vi "Configure System (Beeper).vi"(8 "error in (no error)":errorcluster, 9 "Beeper Tone (3: Tone 3)":u16(ring)=3 items=["Tone 1"=1, "Tone 2"=2, "Tone 3"=3, "Tone 4"=4, "Tone 5"=5], 10 "Beeper State (F:Disable)":bool, 11 "VISA resource name":refnum<visa-resource-name>) -> (0 "error out":errorcluster, 3 "VISA resource name out":refnum<visa-resource-name>)   [LabVIEW 2017, in "Agilent E4980.lvlib"]
doc: "Enables or disables a beeper sound, and selects a beeper sound tone."
uses:
  Agilent E4980.lvlib
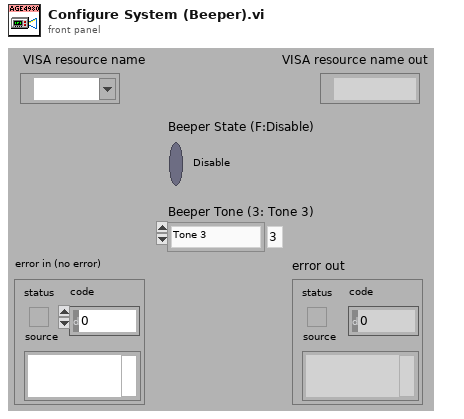
[diagram p1: front panel]
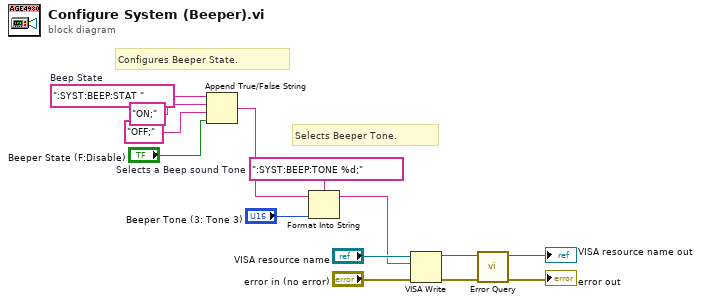
[diagram p0: block diagram]
diagram:
  w10 = ":SYST:BEEP:TONE %d;"  # Selects a Beep sound Tone
  w14 = ":SYST:BEEP:STAT "  # Beep State
  # "Configures Beeper State."
  # "Selects Beeper Tone."
  n1 = Append True/False String(1:"Beeper State (F:Disable)", 2:"OFF;", 3:"ON;" ("true string"), 4:w14) -> (0:w9:string)
  n2 = Format Into String(format string=w10, initial string=w9, "Beeper Tone (3: Tone 3)") -> (resulting string=w6:string)  [unwired: 1 in, 1 out]
  n3 = VISA Write(VISA resource name="VISA resource name", write buffer=w6, error in (no error)="error in (no error)") -> (VISA resource name out=w5:refnum<visa-resource-name>, error out=w4:errorcluster)  [unwired: 1 out]
  n4 = call "Error Query.vi"("error in (no error)"=w4, "VISA resource name"=w5) -> ("error out"=→"error out":errorcluster, "VISA resource name out"=→"VISA resource name out":refnum<visa-resource-name>)  [unwired: 6 in, 2 out]
